vi "GE 5565PIORC.Registers.LIER.Local Memory Parity Error Interrupt Enable.Get.vi"(8 "error in (no error)":errorcluster, 11 "GE 5565PIORC in":refnum<class "GE 5565PIORC.lvclass">) -> (0 "error out":errorcluster, 2 "Local Memory Parity Error Interrupt Enable":bool, 3 "GE 5565PIORC out":refnum<class "GE 5565PIORC.lvclass">)   [LabVIEW 2024, in "GE 5565PIORC.lvclass"]
doc: "Enables or disables the specified interrupt. Each interrupt enable bit corresponds to a status bit in the Local Interrupt Status Register (LISR)."
uses:
  GE 5565PIORC.lvclass
  GE 5565PIORC.Registers.RFM Control and Status.ctl
  GE 5565PIORC.lvclass/GE 5565PIORC.ctl
  GE 5565PIORC.Registers.RFM Control and Status.Read (U32).vi
  Methods/GE 5565PIORC.Bit Manipulation.Get Bit (U32).vi
  Methods/GE 5565PIORC.Registers.Read.vi
  Methods/GE 5565PIORC.Registers.Read (U32).vi
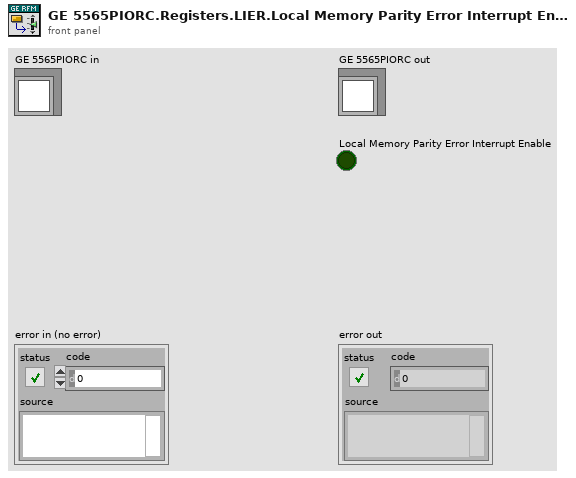
[diagram p1: front panel]
types:
  T1 = typedef "GE 5565PIORC.lvclass/GE 5565PIORC.Registers.RFM Control and Status.ctl" = u32
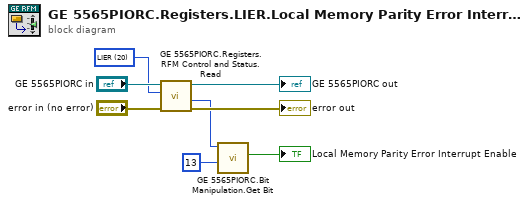
[diagram p0: block diagram]
diagram:
  w4 = T1 20 items=["BRV"=0, "BID"=1, "BRB"=2, "NID"=4, "LCSR1"=8, "LISR"=16, "LIER"=20, "NTD"=24, "NTN"=28, "NIC"=29, "ISD1"=32, "SID1"=36, "ISD2"=40, "SID2"=44, "ISD3"=48, "SID3"=52, "ISD4"=56, "SID4"=60] ("Register")
  n1 = call-poly "GE 5565PIORC.Registers.RFM Control and Status.Read.vi"("error in (no error)"="error in (no error)", "Register"=w4, "GE 5565PIORC in"="GE 5565PIORC in") -> ("error out"=→"error out":errorcluster, "Value"=w3:u32, "GE 5565PIORC out"=→"GE 5565PIORC out":refnum<class "GE 5565PIORC.lvclass">)  [unwired: 6 in]
  n2 = call-poly "GE 5565PIORC.Bit Manipulation.Get Bit.vi"("bit index"=13, "packed value in"=w3) -> ("bit"=→"Local Memory Parity Error Interrupt Enable":bool)  [unwired: 8 in, 1 out]
